vi "Destroy.vi"(8 "error in (no error)":errorcluster, 11 "CIF_DAQ_DVR_Multi in":refnum<class "CIF_NIChn_DAQ.lvclass">) -> (0 "error out":errorcluster, 3 "CIF_DAQ_DVR_Multi out":refnum<class "CIF_NIChn_DAQ.lvclass">)   [LabVIEW 2021, in "CIF_NIChn_DAQ.lvclass"]
uses:
  CIF_NIChn_DAQ.lvclass
  D:/dev/Packages/Channel_Manager/src/CIFChannels/CIFChannels.lvclass
  CIFChannels/CIFChannels.lvclass/CIFChannels.ctl
  CIF_NIChn_DAQ.lvclass/CIF_NIChn_DAQ.ctl
  DAQ Base/CIF_NIChn_DAQ_Base.lvclass
  CIFChannels/CIFChannels.lvclass
  D:/dev/Packages/Channel_Manager/src/CIF_NIChn/FIFO_DAQ/DAQ Base/CIF_NIChn_DAQ_Base.lvclass
  D:/dev/Packages/Channel_Manager/src/CIF_NIChn/FIFO_U8/CIF_NIChn_Fifo_U8.lvclass
  D:/dev/Packages/Channel_Manager/src/CIF_NIChn/NIChn/CIF_NIChn.lvclass
  D:/dev/Packages/Channel_Manager/src/CIF_NIChn/FIFO_DAQ/CIF_NIChn_DAQ.lvclass
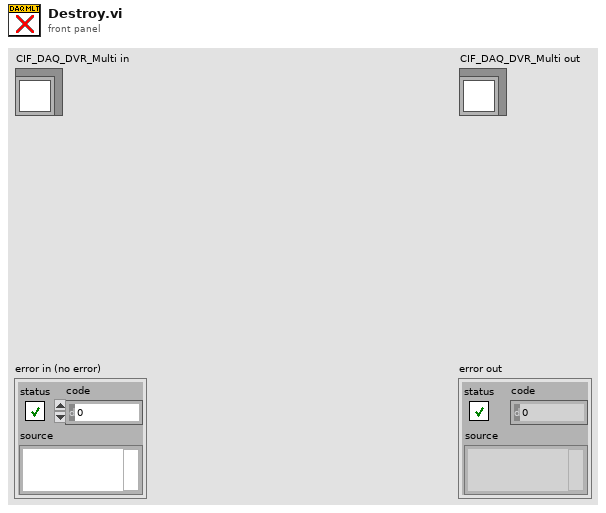
[diagram p1: front panel]
types:
  T1 = typedef "CIFChannels.lvclass/Direction.ctl" = enum16{"Publisher", "Subscriber"}
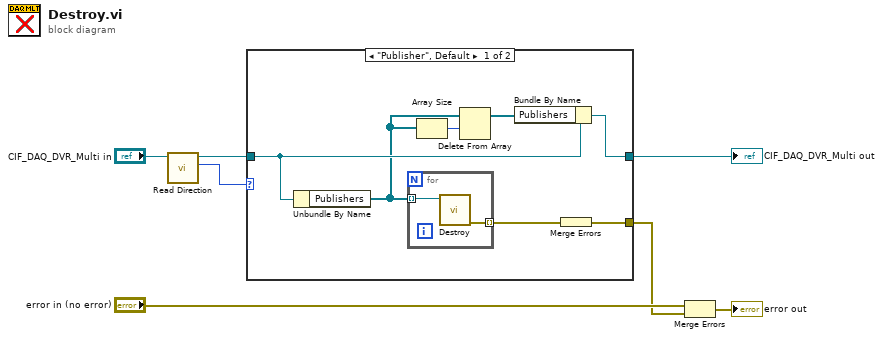
[diagram p0: block diagram]
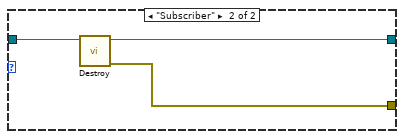
[diagram p2: hidden frame]
diagram:
  n1 = call "Read Direction.vi"("CIFChannels in"="CIF_DAQ_DVR_Multi in") -> ("Direction"=w6:T1, "CIFChannels out"=w5:refnum<class "CIF_NIChn_DAQ.lvclass">)  [unwired: 8 in, 1 out]
  n2 = case shown="\"Publisher\", Default" w6 {
    tunnel: w5 -> [w14 w19]
    tunnel: [w11 w17] -> w2
    tunnel: [w13 w18] -> w4
    frame "Publisher", Default {
      n3 = Unbundle By Name(w14) -> ("Publishers"=w9:refnum<class "CIF_NIChn_DAQ_Base.lvclass">[])
      n4 = for {
        tunnel: w9 -> [w16] mode=indexing
        tunnel: [w15] -> w12 mode=indexing
        n5 = call-dynamic "Destroy.vi"("CIF_NIChn_FIFO_DAQ in"=w16) -> ("error out"=w15:errorcluster)  [unwired: 9 in, 1 out]
      }
      n6 = Array Size(array=w9) -> (size(s)=w10:i32)
      n7 = Delete From Array(array=w9, length=w10) -> (array with subset deleted=w8:refnum<class "CIF_NIChn_DAQ_Base.lvclass">[])  [unwired: 1 in, 1 out]
      n8 = Bundle By Name(cluster=w14, "Publishers"=w8) -> (w13:refnum<class "CIF_NIChn_DAQ.lvclass">)
      n9 = Merge Errors(w12) -> (w11:errorcluster)
    }
    frame "Subscriber" {
      n10 = call-parent "Destroy.vi"("CIF_NIChn_FIFO_DAQ in"=w19) -> ("error out"=w17:errorcluster, "CIF_NIChn_FIFO_DAQ out"=w18:refnum<class "CIF_NIChn_DAQ.lvclass">)  [unwired: 9 in]
    }
  }
  "CIF_DAQ_DVR_Multi out" <- w4
  n11 = Merge Errors("error in (no error)", w2) -> (→"error out":errorcluster)
